vi "AutoGenerateAngles.vi"(5 "Randomization Reset":dbl=100.0 format="%#_13g") -> (4 "Value":dbl)   [LabVIEW 2021]
uses:
  <vilib>/numeric/Random Number (Range) DBL.vi
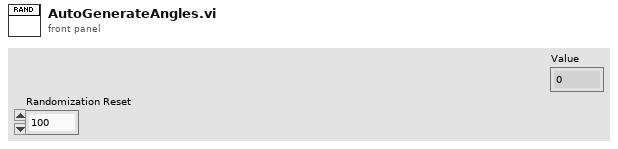
[diagram p1: front panel]
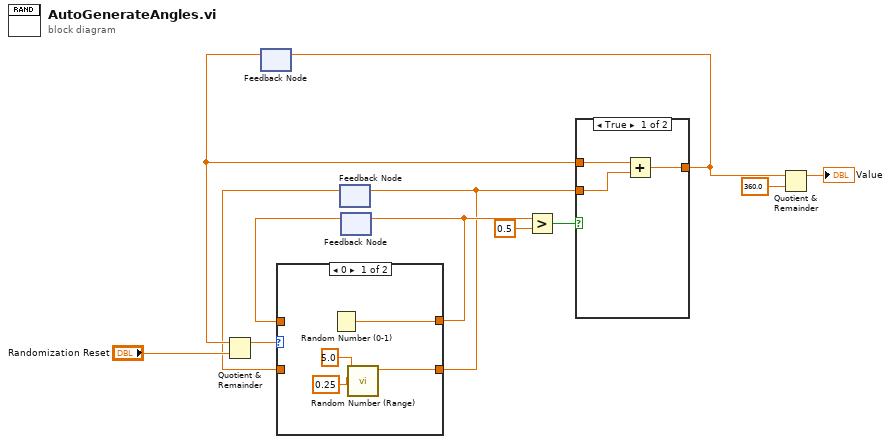
[diagram p0: block diagram]
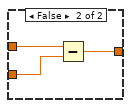
[diagram p3: hidden frame]
diagram:
  n1 = feedback #1() -> (w7:dbl)  [unwired: 1 in]
  n2 = Quotient & Remainder(x=w7, y="Randomization Reset") -> (x-y*floor(x/y)=w5:dbl)  [unwired: 1 out]
  n3 = feedback #2() -> (w2:dbl)  [unwired: 1 in]
  n4 = feedback #3() -> (w4:dbl)  [unwired: 1 in]
  n5 = case shown="0" w5 {
    tunnel: [w16 w18] -> w3
    tunnel: w4 -> [_ w18]
    tunnel: [w13 w17] -> w1
    tunnel: w2 -> [_ w17]
    frame 0 {
      n6 = Random Number (0-1)() -> (number: 0 to 1=w16:dbl)
      n7 = call-poly <vilib>:"Random Number (Range).vi"("lower bound (0)"=0.25, "upper bound (100)"=5.0) -> ("number"=w13:dbl)  [unwired: 9 in]
    }
    frame Default {
    }
  }
  n8 = feedback-in #2(w1) -> ()
  n9 = feedback-in #3(w3) -> ()
  n10 = Greater?(x=w3, y=0.5) -> (0:w9:bool)
  n11 = case shown="True" w9 {
    tunnel: w7 -> [w21 w24]
    tunnel: w1 -> [w20 w23]
    tunnel: [w19 w22] -> w12
    frame True {
      n12 = Add(x=w21, y=w20) -> (x+y=w19:dbl)
    }
    frame False {
      n13 = Subtract(x=w24, y=w23) -> (x-y=w22:dbl)
    }
  }
  n14 = feedback-in #1(w12) -> ()
  n15 = Quotient & Remainder(x=w12, y=360.0) -> (x-y*floor(x/y)=→"Value":dbl)  [unwired: 1 out]
